vi "RectCentroid.vi"(8 "错误输入":errorcluster, 11 "Rect In":T1 caption="矩形") -> (0 "错误输出":errorcluster, 2 "point":cluster{"x":i16, "y":i16} caption="点", 3 "Rect Out":T1 caption="矩形")   [LabVIEW 2012, in "Rect Tools.lvlib"]
uses:
  Rect Tools.lvlib
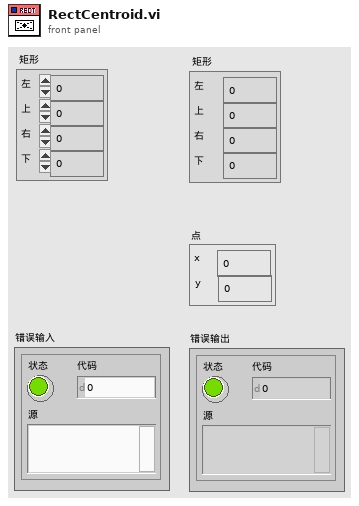
[diagram p1: front panel]
types:
  T1 = cluster{"left":i16, "top":i16, "right":i16, "bottom":i16}
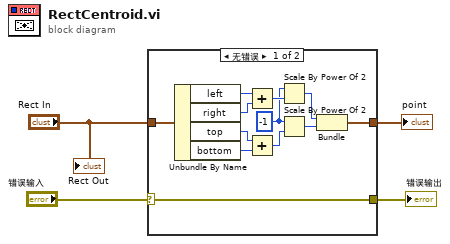
[diagram p0: block diagram]
diagram:
  n1 = case shown="无错误" "错误输入" {
    selector: "错误输入" -> [w7 w17]
    tunnel: [w7 w17] -> w3
    tunnel: "Rect In" -> [w6 _]
    tunnel: [w5 _] -> w2
    frame No Error {
      w10 = -1
      n2 = Unbundle By Name(w6) -> ("left"=w16:i16, "right"=w15:i16, "top"=w14:i16, "bottom"=w13:i16)
      n3 = Add(x=w16, y=w15) -> (x+y=w11:i16)
      n4 = Add(x=w14, y=w13) -> (x+y=w12:i16)
      n5 = Scale By Power Of 2(n=w10, x=w11) -> (x*2^n=w9:i16)
      n6 = Scale By Power Of 2(n=w10, x=w12) -> (x*2^n=w8:i16)
      n7 = Bundle(w9, w8) -> (w5:cluster{i16, i16})  [unwired: 1 in]
    }
    frame Error {
    }
  }
  "错误输出" <- w3
  "point" <- w2
  "Rect Out" <- "Rect In"
